vi "Window_Avg_and_Spark_Rate_Median.vi"(3 "Window size [min]":i64=5 min=1 max=180, 4 "Threshold":dbl, 5 "Current in":dbl[](array[numeric])) -> (0 "Window Spark Rate":dbl, 1 "Window Avg":dbl, 2 "window median":dbl format="%0.2f")   [LabVIEW 2018]
uses:
  <vilib>/Analysis/NI_AALBase.lvlib
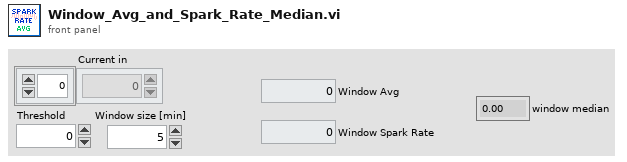
[diagram p1: front panel]
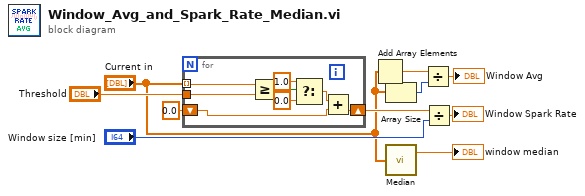
[diagram p0: block diagram]
diagram:
  n1 = for {
    tunnel: "Current in" -> [w18] mode=indexing
    shift-right: [w14] -> w7
    shift-left: 0.0 ("f") -> [w12]
    tunnel: "Threshold" -> [w11]
    n2 = Greater Or Equal?(x=w18, y=w11) -> (x >= y?=w17:bool)
    n3 = Select(t=1.0, s=w17, f=0.0) -> (s? t:f=w15:dbl)
    n4 = Add(x=w15, y=w12) -> (x+y=w14:dbl)
  }
  n5 = Add Array Elements(numeric array="Current in") -> (sum=w8:dbl)
  n6 = Array Size(array="Current in") -> (size(s)=w9:i32)
  n7 = call <vilib>:"Median.vi"("X"="Current in") -> ("median"=→"window median":dbl)  [unwired: 1 out]
  n8 = Divide(x=w8, y=w9) -> (x/y=→"Window Avg":dbl)
  n9 = Divide(x=w7, y="Window size [min]") -> (x/y=→"Window Spark Rate":dbl)
